vi "Write DML Global.vi"(10 "DriveMotorsLeft.lvclass":refnum<class "DriveMotorsLeft.lvclass">) -> ()   [LabVIEW 2013]
uses:
  DriveMotorsLeft.lvclass
  Robot Global Data.vi
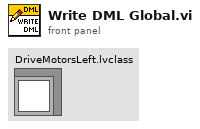
[diagram p1: front panel]
types:
  T1 = typedef "Semaphore RefNum" = refnum<k1>
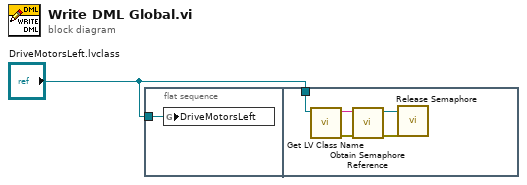
[diagram p0: block diagram]
diagram:
  n1 = flat-sequence {
    tunnel: "DriveMotorsLeft.lvclass" -> [w2]
    tunnel: "DriveMotorsLeft.lvclass" -> [w6]
    frame #0 {
      n2 = global write "Robot Global Data.vi" "DriveMotorsLeft"(w2) -> ()
    }
    frame #1 {
      n3 = call <vilib>:"Get LV Class Name.vi"("object"=w6) -> ("error out"=w3:errorcluster, "class name"=w7:string)  [unwired: 9 in]
      n4 = call <vilib>:"Obtain Semaphore Reference.vi"("error in (no error)"=w3, "name (unnamed)"=w7) -> ("error out"=w5:errorcluster, "semaphore"=w4:T1)  [unwired: 3 in, 1 out]
      n5 = call <vilib>:"Release Semaphore.vi"("error in (no error)"=w5, "semaphore"=w4) -> ()  [unwired: 4 in, 2 out]
    }
  }
